vi "read_return.vi"(3 "错误输入（无错误）":errorcluster, 5 "com in":refnum<visa-resource-name>) -> (0 "错误输出":errorcluster, 1 "return out":u8[](array[numeric]), 2 "com out":refnum<visa-resource-name>)   [LabVIEW 2018]
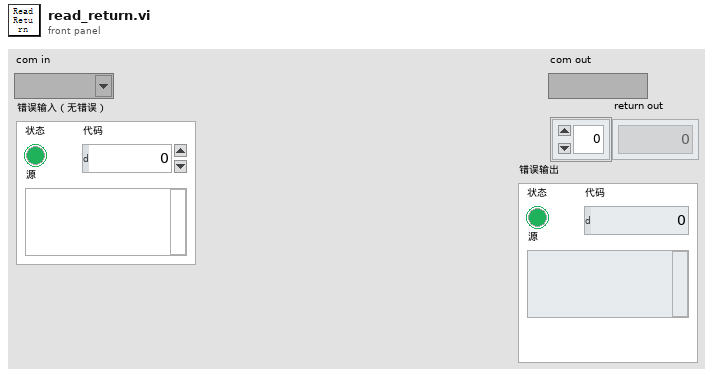
[diagram p1: front panel]
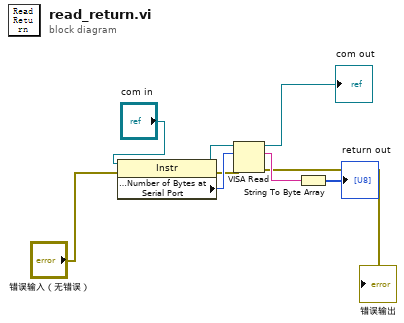
[diagram p0: block diagram]
diagram:
  n1 = property class="Instr"(reference="com in", error in="错误输入（无错误）") -> (reference out=w6:refnum<visa-resource-name>, error out=w1:errorcluster, "Serial Settings:Number of Bytes at Serial Port"=w7:u32)
  n2 = VISA Read(VISA resource name=w6, byte count=w7, error in (no error)=w1) -> (VISA resource name out=→"com out":refnum<visa-resource-name>, read buffer=w5:string, error out=→"错误输出":errorcluster)  [unwired: 1 out]
  n3 = String To Byte Array(string=w5) -> (unsigned byte array=→"return out":u8[])
